vi "DBCatchLED.vi"(9 "Catch":bool, 10 "DBNames":string[](array[string]), 11 "PulsePeriod(ms)":u16=500) -> ()   [LabVIEW 2016]
uses:
  <vilib>/Rock Robotics/Network Tables/NT Write Boolean.vi
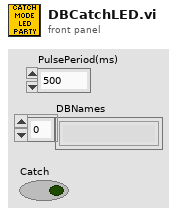
[diagram p1: front panel]
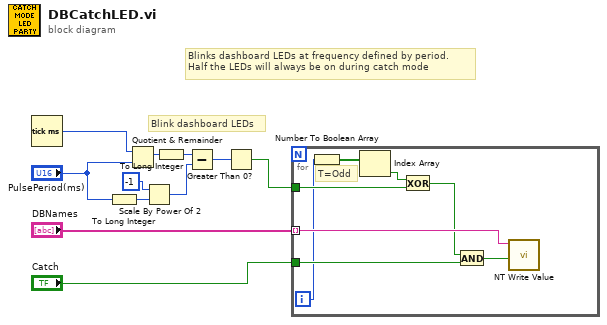
[diagram p0: block diagram]
diagram:
  # "Blinks dashboard LEDs at frequency defined by period.\nHalf the LEDs will always be on during catch mode"
  # "Blink dashboard LEDs"
  n1 = Tick Count (ms)() -> (millisecond timer value=w10:u32)
  n2 = To Long Integer(number="PulsePeriod(ms)") -> (32bit integer=w4:i32)
  n3 = Quotient & Remainder(x=w10, y="PulsePeriod(ms)") -> (x-y*floor(x/y)=w9:u32)  [unwired: 1 out]
  n4 = Scale By Power Of 2(n=i16 -1, x=w4) -> (x*2^n=w5:i32)
  n5 = To Long Integer(number=w9) -> (32bit integer=w8:i32)
  n6 = Subtract(x=w8, y=w5) -> (x-y=w3:i32)
  n7 = Greater Than 0?(x=w3) -> (x > 0?=w2:bool)
  n8 = for {
    tunnel: "DBNames" -> [w19] mode=indexing
    tunnel: w2 -> [w16]
    tunnel: "Catch" -> [w14]
    i -> [w12]
    # "T=Odd"
    n9 = Number To Boolean Array(number=w12) -> (Boolean array=w18:bool[])
    n10 = Index Array(array=w18) -> (element=w17:bool)  [unwired: 1 in]
    n11 = Exclusive Or(1:w16, 2:w17) -> (0:w15:bool)
    n12 = And(x=w15, y=w14) -> (x .and. y?=w13:bool)
    n13 = call-poly <vilib>:"NT Write Value.vi"("Boolean"=w13, "Name"=w19) -> ()  [unwired: 9 in, 1 out]
  }
